vi "write_data_to_fpga.vi"   [LabVIEW 2017, in "fpga_interface.lvlib"]
uses:
  fpga_interface.lvlib
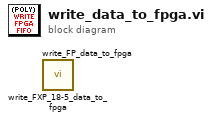
[diagram p0: block diagram]
diagram:
  n1 = call "write_FXP_18-5_data_to_fpga.vi"() -> ()  [unwired: 10 in, 2 out]
  n2 = call "write_FP_data_to_fpga.vi"() -> ()  [unwired: 10 in, 2 out]
